vi "Get Toolkit Used List.vi"(10 "Version":string, 11 "Exe License Path":path) -> (0 "error out":errorcluster, 3 "Open Source Toolkit Used":string[](array[string]))   [LabVIEW 2020]
uses:
  <userlib>/_OpenG.lib/lvzip/lvzip.llb/ZLIB Extract File__ogtk.vi
  <userlib>/_OpenG.lib/lvzip/lvzip.llb/ZLIB Open Unzip Archive__ogtk.vi
  <vilib>/JKI/VIPM API/VIPM API_vipm_api.lvlib
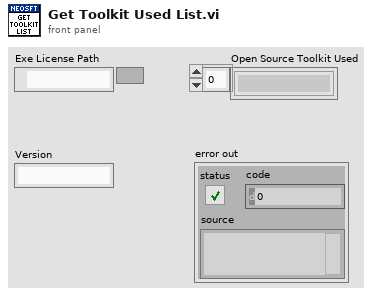
[diagram p1: front panel]
types:
  T1 = typedef "VIPM API_vipm_api.lvlib/Library Contents Cluster_vipm_api.ctl" = cluster{"Package Name":string, "Version":string, "Display Name":string, "Repository Name":string, "Company Name":string, "License Type":string, "Installed":bool, "Deprecated":bool, "Dependency or Conflict Problem":bool, "Downloaded":bool}
  T2 = typedef "ZLIB Unzip Handle__ogtk.ctl" = refnum<k1>
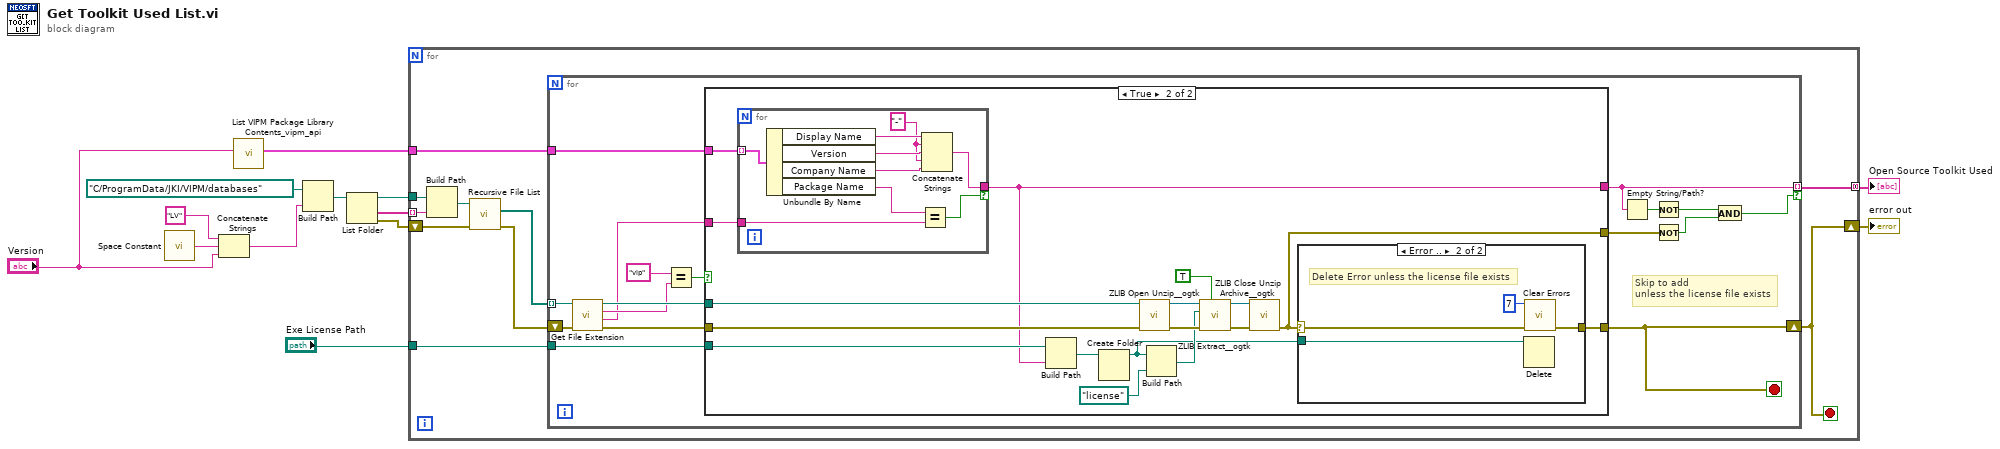
[diagram p0: block diagram]
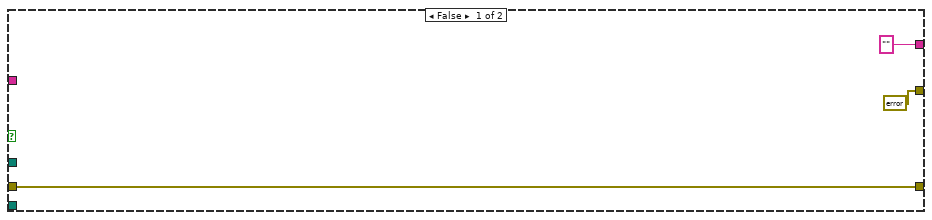
[diagram p2: hidden frame]
diagram:
  n1 = call <vilib>:"Space Constant.vi"() -> ("String"=w5:string)
  n2 = Concatenate Strings("LV" ("string"), w5, "Version") -> (w3:string)
  n3 = call <vilib>:"List VIPM Package Library Contents_vipm_api.vi"("LabVIEW Version"="Version") -> ("Library Contents []"=w12:T1[])  [unwired: 8 in, 2 out]
  n4 = Build Path(base path=path "C:/ProgramData/JKI/VIPM/databases", name or relative path=w3) -> (appended path=w6:path)
  n5 = List Folder(path=w6) -> (path out=w7:path, folder names=w8:string[], error out=w9:errorcluster)  [unwired: 3 in, 1 out]
  n6 = for {
    tunnel: w7 -> [w23]
    tunnel: w8 -> [w22] mode=indexing
    shift-right: [w17] -> w1
    shift-left: w9 -> [w19]
    tunnel: "Exe License Path" -> [w16]
    tunnel: w12 -> [w15]
    tunnel: [w14] -> w13 mode=concatenating
    stop <- w17 stop-if-true
    n7 = Build Path(base path=w23, name or relative path=w22) -> (appended path=w21:path)
    n8 = call <vilib>:"Recursive File List.vi"("error in (no error)"=w19, "Folder Path"=w21) -> ("error out"=w18:errorcluster, "All Files in Dir"=w20:path[])  [unwired: 5 in, 3 out]
    n9 = for {
      tunnel: w20 -> [w40] mode=indexing
      shift-right: [w35] -> w17
      shift-left: w18 -> [w37]
      tunnel: w16 -> [w28]
      tunnel: w15 -> [w32]
      tunnel: [w30] -> w14 mode=indexing if=w26
      stop <- w35 stop-if-true
      # "Skip to add\nunless the license file exists"
      n10 = call <vilib>:"Get File Extension.vi"("error in (no error)"=w37, "file"=w40) -> ("error out"=w36:errorcluster, "filename without extension"=w31:string, "lowercase file extension"=w33:string, "dup file"=w38:path)  [unwired: 5 in, 1 out]
      n11 = Equal?(x="vip" ("y"), y=w33) -> (x = y?=w39:bool)
      n12 = case shown="True" w39 {
        tunnel: w38 -> [_ w60]
        tunnel: w36 -> [w43 w57]
        tunnel: [w43 w46] -> w35
        tunnel: w32 -> [_ w51]
        tunnel: w31 -> [_ w50]
        tunnel: ["" ("Display Name") w47] -> w30
        tunnel: w28 -> [_ w49]
        tunnel: [errorcluster {"status"=FALSE, "code"=0, "source"=""} ("error out") w44] -> w24
        frame False {
        }
        frame True {
          n13 = for {
            tunnel: w51 -> [w74] mode=indexing
            tunnel: w50 -> [w73]
            tunnel: [w66] -> w47 if=w72
            w68 = "-"
            n14 = Unbundle By Name(w74) -> ("Display Name"=w70:string, "Version"=w69:string, "Company Name"=w67:string, "Package Name"=w71:string)
            n15 = Equal?(x=w71, y=w73) -> (x = y?=w72:bool)
            n16 = Concatenate Strings(w70, w68, w69, w68, w67) -> (w66:string)
          }
          n17 = Build Path(base path=w49, name or relative path=w47) -> (appended path=w48:path)
          n18 = Create Folder(path (use dialog)=w48) -> (created path=w45:path)  [unwired: 2 in, 2 out]
          n19 = call-poly <userlib>:"ZLIB Open Unzip__ogtk.vi"("error in (no error)"=w57, "archive name"=w60) -> ("error out"=w55:errorcluster, "unzip Refnum"=w54:T2)  [unwired: 4 in]
          n20 = Build Path(base path=w45, name or relative path=path "license") -> (appended path=w52:path)
          n21 = call-poly <userlib>:"ZLIB Extract__ogtk.vi"("overwrite (F)"=TRUE, "error in (no error)"=w55, "target path"=w52, "unzip Refnum"=w54) -> ("error out"=w58:errorcluster, "unzip Refnum out"=w59:T2)  [unwired: 4 in]
          n22 = call <userlib>:"ZLIB Close Unzip Archive__ogtk.vi"("error in (no error)"=w58, "unzip Refnum"=w59) -> ("error out"=w44:errorcluster)  [unwired: 5 in]
          n23 = case shown="Error .." w44 {
            selector: w44 -> [w61 w65]
            tunnel: [w61 w64] -> w46
            tunnel: w45 -> [_ w63]
            frame No Error {
            }
            frame Error {
              # "Delete Error unless the license file exists"
              n24 = Delete(path (use dialog)=w63) -> ()  [unwired: 4 in, 3 out]
              n25 = call <vilib>:"Clear Errors.vi"("error in (no error)"=w65, "specific error code to clear (0: all)"=7) -> ("error out"=w64:errorcluster)  [unwired: 4 in, 1 out]
            }
          }
        }
      }
      n26 = Empty String/Path?(string/path=w30) -> (empty?=w29:bool)
      n27 = Not(x=w29) -> (.not. x?=w27:bool)
      n28 = Not(x=w24) -> (.not. x?=w25:bool)
      n29 = And(x=w27, y=w25) -> (x .and. y?=w26:bool)
    }
  }
  "Open Source Toolkit Used" <- w13
  "error out" <- w1
